vi "Async Loop.vi"(8 "error in (no error)":errorcluster, 10 "Process Data":T2, 11 "Path":path) -> (0 "error out":errorcluster)   [LabVIEW 2020, in "Shared Variables CD 2.0 Engine.lvlib"]
uses:
  Shared Variables CD 2.0 Engine.lvlib
  <vilib>/NI VeriStand/Custom Device Tools/Custom Device Utility Library/Custom Device Utility Library.lvlib
  Shared DataTypes/URLs.ctl
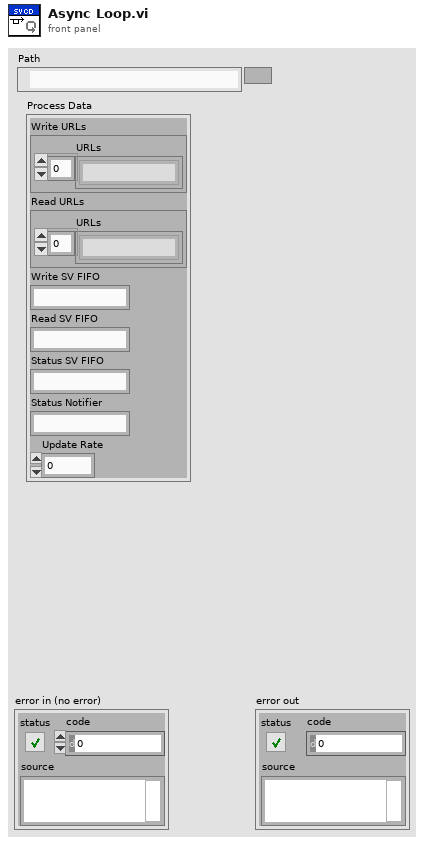
[diagram p1: front panel]
types:
  T1 = typedef "URLs.ctl" = cluster{"URLs":string[]}
  T2 = cluster{"Write URLs":T1, "Read URLs":T1, "Write SV FIFO":string, "Read SV FIFO":string, "Status SV FIFO":string, "Status Notifier":string, "Update Rate":u32}
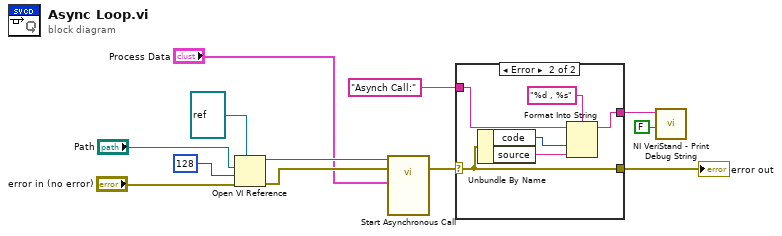
[diagram p0: block diagram]
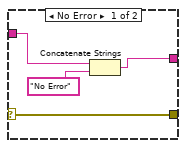
[diagram p2: hidden frame]
diagram:
  n1 = Open VI Reference(type specifier VI Refnum (for type only)=refnum<vi> refnum, vi path="Path", options=128, error in (no error)="error in (no error)") -> (vi reference=w2:refnum<vi>, error out=w5:errorcluster)  [unwired: 2 in]
  n2 = call-by-ref "Start Asynchronous Call"(reference=w2, error in=w5, "Process Data"="Process Data") -> (error out=w4:errorcluster)  [unwired: 9 in, 2 out]
  n3 = case shown="Error" w4 {
    selector: w4 -> [w16 w21]
    tunnel: [w16 w21] -> w10
    tunnel: "Asynch Call:" ("Message") -> [w15 w22]
    tunnel: [w13 w17] -> w8
    frame No Error {
      n4 = Concatenate Strings(w15, "No Error" ("string")) -> (w13:string)
    }
    frame Error {
      n5 = Unbundle By Name(w21) -> ("code"=w20:i32, "source"=w19:string)
      n6 = Format Into String(format string="%d , %s", initial string=w22, w20, w19) -> (resulting string=w17:string)  [unwired: 1 in, 1 out]
    }
  }
  "error out" <- w10
  n7 = call <vilib>:"NI VeriStand - Print Debug String.vi"("Add to log file? (F)"=FALSE ("Add to log file? (T)"), "Message"=w8) -> ()  [unwired: 9 in, 1 out]
